vi "Initialize.vi"(8 "error in":errorcluster, 10 "settings in":T2, 11 "Device Reference in":T3 format="%.0x") -> (0 "error out":errorcluster, 1 "inline runtime data":T1, 2 "settings out":T2, 3 "Device Reference out":T3 format="%.0x")   [LabVIEW 2019, in "HLA Custom Device Engine.lvlib"]
uses:
  HLA Custom Device Engine.lvlib
  <vilib>/NI VeriStand/Custom Device API/Custom Device Item Ref.ctl
  Shared/Compiled.Settings.ctl
  RTinlineRuntimeData.ctl
  <vilib>/NI VeriStand/Custom Device API/Custom Device API.lvlib
  Shared/HLA Custom Device Shared.lvlib
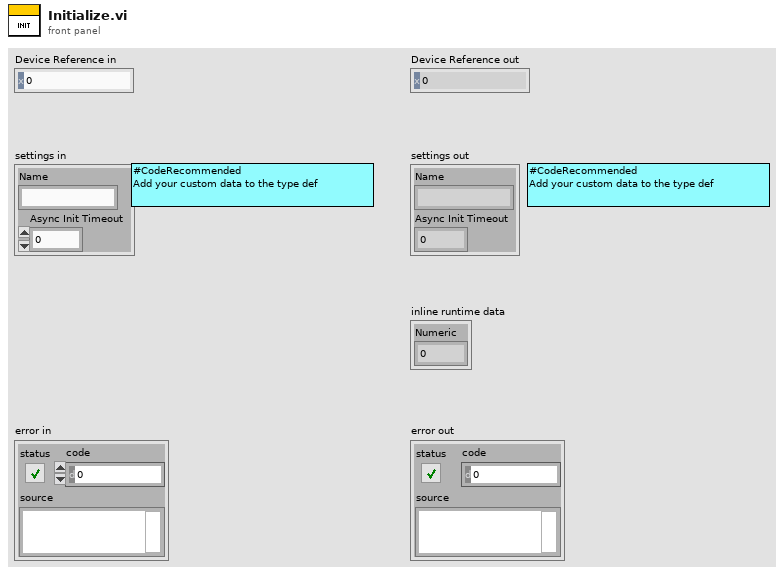
[diagram p1: front panel]
types:
  T1 = typedef "HLA Custom Device Engine.lvlib/RTinlineRuntimeData.ctl" = cluster{"Numeric":dbl}
  T2 = typedef "HLA Custom Device Shared.lvlib/Compiled.Settings.ctl" = cluster{"Name":string, "Async Init Timeout":u16}
  T3 = typedef "Custom Device API.lvlib/Custom Device Item Ref.ctl" = u64
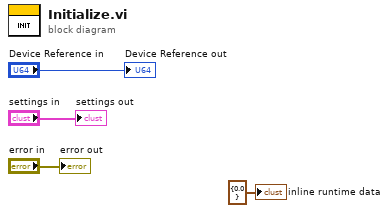
[diagram p0: block diagram]
diagram:
  "Device Reference out" <- "Device Reference in"
  "settings out" <- "settings in"
  "error out" <- "error in"
  "inline runtime data" <- T1 {"Numeric"=0.0} ("inline runtime data")
